vi "test insert_component.vi"() -> ()   [LabVIEW 2023]
uses:
  DB Component.ctl
  Database.lvlib
panel:
  out "Component out":T1
  out "error out":errorcluster
  in  "port":i32=33060
  in  "host":string="localhost"
  in  "password":string="carriker"
  in  "username":string="root"
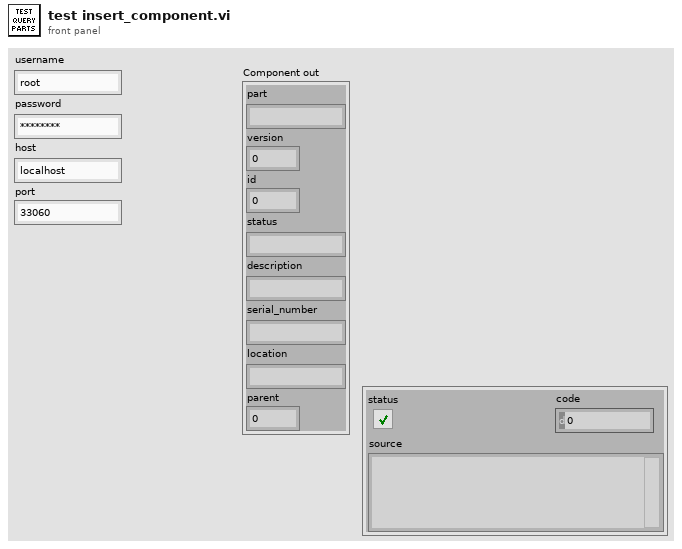
[diagram p1: front panel]
types:
  T1 = typedef "Database.lvlib/DB Component.ctl" = cluster{"part":string, "version":i32, "id":i32, "status":string, "description":string, "serial_number":string, "location":string, "parent":i32}
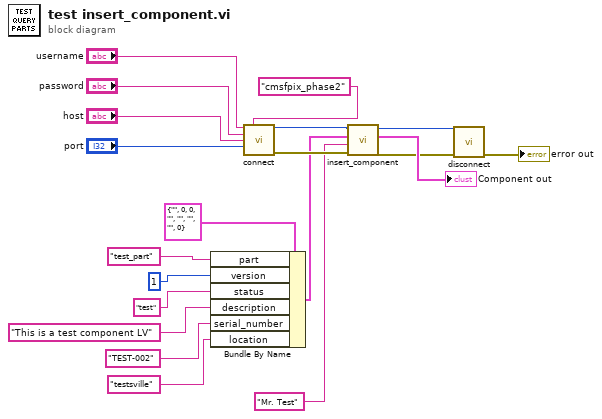
[diagram p0: block diagram]
diagram:
  n1 = Bundle By Name(cluster=T1 {"part"="", "version"=0, "id"=0, "status"="", "description"="", "serial_number"="", "location"="", "parent"=0} ("Component"), "part"="test_part", "version"=1, "status"="test", "description"="This is a test component LV", "serial_number"="TEST-002", "location"="testsville") -> (w2:T1)
  n2 = call "connect.vi"("username"="username", "schema"="cmsfpix_phase2" ("Schema"), "password"="password", "host"="host", "port"="port") -> ("DB Session ID"=w15:i32, "error out"=w14:errorcluster)  [unwired: 9 in]
  n3 = call "insert_component.vi"("error in (no error)"=w14, "who"="Mr. Test", "Component"=w2, "DB Session ID"=w15) -> ("error out"=w11:errorcluster, "Component out"=→"Component out":T1, "DB Session ID out"=w12:i32)  [unwired: 5 in]
  n4 = call "disconnect.vi"("DB Session ID"=w12, "error in (no error)"=w11) -> ("error out"=→"error out":errorcluster)  [unwired: 13 in]
